vi "Start Logic-Mode dependent case 1.vi"(6 "Case name string":string, 8 "error in (no error)":errorcluster, 11 "UI queue":refnum<queue>) -> (0 "error out":errorcluster)   [LabVIEW 2013]
uses:
  Queue/Message Queue/Typedefs/Message Cluster.ctl
  Global Variables/gl_UI Ctrl Refs.vi
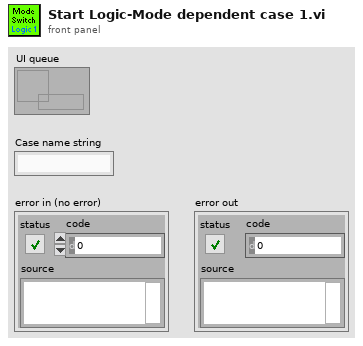
[diagram p1: front panel]
types:
  T1 = typedef "UI ctrl refs cluster.ctl" = cluster{"Top level VI path":path, "Top level VI ref":refnum<vi>, "User menu ref":refnum<k9>, "Sub Panel control":refnum<vi>, "Imaging Param Tab":refnum<vi>, "Occurrence-Start drivers":refnum<k4>, "Occurrence-Speed logging initialised":refnum<k4>, "Occurrence-XYZ stage initialised":refnum<k4>, "Exit button":refnum<vi>, "Status ind":refnum<vi>, "Return to Origin":refnum<vi>, "Speed Logging":refnum<vi>, "Time Lapse":refnum<vi>, "Live Imaging":refnum<vi>, "AOL Z Stack":refnum<vi>, "Motor Z Stack":refnum<vi>, "Funct Acq button":refnum<vi>, "Hard Shutter":refnum<vi>, "Virtual Shutter":refnum<vi>, "Laser Power":refnum<vi>, "AOL Mode":refnum<vi>, "Frame Size":refnum<vi>, "Field of View":refnum<vi>, "Dwell Time":refnum<vi>, "Zoom":refnum<vi>, "AOL Z":refnum<vi>, "Objective":refnum<vi>, "Axis":refnum<vi>, "Paths & Names":refnum<vi>, "Experiment folder path (ind.)":refnum<vi>, "Last State (Ind.)":refnum<vi>, "Laser wavelength ind (nm)":refnum<vi>, "Averages":refnum<vi>, "Angle (degrees)":refnum<vi>, "X centre":refnum<vi>, "Y centre":refnum<vi>, "Plane Mode":refnum<vi>, "# Planes":refnum<vi>, "Z Start":refnum<vi>, "Z Stop":refnum<vi>, "Z Step":refnum<vi>, "PMT 1":refnum<vi>, "PMT 2":refnum<vi>, "Stage XYZ Position":refnum<vi>, "Pockels@Z Start":refnum<vi>, "Pockels@Z Stop":refnum<vi>, "Obtain Z Start":refnum<vi>, "Obtain Z Stop":refnum<vi>, "Live stim.trig.period":refnum<vi>, "Live stim.trig.enable":refnum<vi>, "Funct. Acq. Pockels Modulation":refnum<vi>, "Enable Video Recording":refnum<vi>, "Video Record-Live Imaging":refnum<vi>, "Video Record-Funct acq":refnum<vi>, "AOL Z-stack Chirps Ready (ind)":refnum<vi>, "Center freq ind (nm)":refnum<vi>, "Logging queue (ind)":refnum<vi>, "Back aperture power (ind.)":refnum<vi>, "Power after objective (ind.)":refnum<vi>, "Switch user":refnum<vi>}
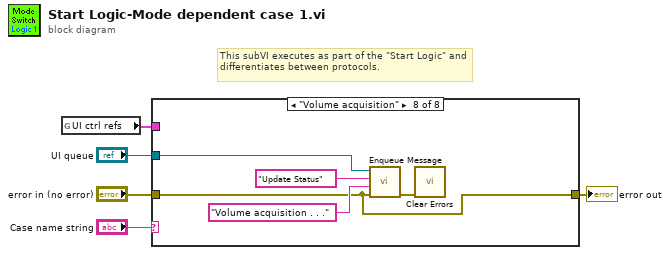
[diagram p0: block diagram]
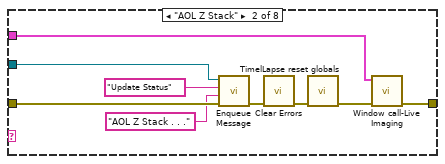
[diagram p3: hidden frame]
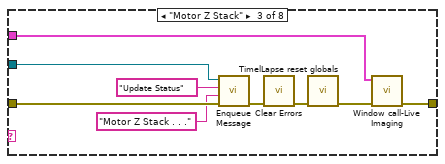
[diagram p4: hidden frame]
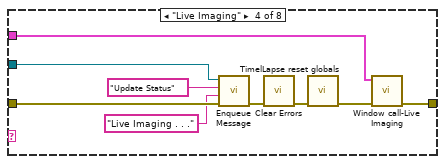
[diagram p5: hidden frame]
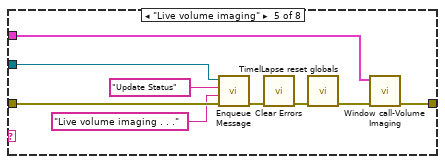
[diagram p6: hidden frame]
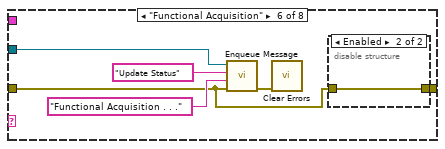
[diagram p7: hidden frame]
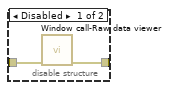
[diagram p8: hidden frame]
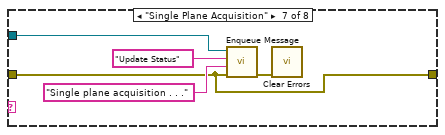
[diagram p9: hidden frame]
diagram:
  # "This subVI executes as part of the \"Start Logic\" and differentiates between protocols."
  n1 = global read "gl_UI Ctrl Refs.vi" "UI ctrl refs"() -> (w2:T1)
  n2 = case shown="\"Volume acquisition\"" "Case name string" {
    tunnel: "error in (no error)" -> [w6 w15 w24 w33 w42 w44 w52 w57]
    tunnel: "UI queue" -> [_ w14 w23 w32 w41 w48 w56 w61]
    tunnel: w2 -> [_ w8 w17 w26 w35 _ _ _]
    tunnel: [w6 w7 w16 w25 w34 w43 w52 w57] -> w1
    frame Default {
    }
    frame "AOL Z Stack" {
      n3 = call "Enqueue Message.vi"("error in (no error)"=w15, "Message Data"="AOL Z Stack . . ." ("Acquiring and Logging..."), "Message"="Update Status", "Queue"=w14) -> ("error out"=w12:errorcluster)  [unwired: 6 in, 1 out]
      n4 = call <vilib>:"Clear Errors.vi"("error in (no error)"=w12) -> ("error out"=w10:errorcluster)  [unwired: 6 in]
      n5 = call "TimelLapse reset globals.vi"("error in (no error)"=w10) -> ("error out"=w9:errorcluster)  [unwired: 10 in]
      n6 = call "Window call-Live Imaging.vi"("error in (no error)"=w9, "UI ctrl refs"=w8) -> ("error out"=w7:errorcluster)  [unwired: 9 in]
    }
    frame "Motor Z Stack" {
      n7 = call "Enqueue Message.vi"("error in (no error)"=w24, "Message Data"="Motor Z Stack . . ." ("Acquiring and Logging..."), "Message"="Update Status", "Queue"=w23) -> ("error out"=w21:errorcluster)  [unwired: 6 in, 1 out]
      n8 = call <vilib>:"Clear Errors.vi"("error in (no error)"=w21) -> ("error out"=w19:errorcluster)  [unwired: 6 in]
      n9 = call "TimelLapse reset globals.vi"("error in (no error)"=w19) -> ("error out"=w18:errorcluster)  [unwired: 10 in]
      n10 = call "Window call-Live Imaging.vi"("error in (no error)"=w18, "UI ctrl refs"=w17) -> ("error out"=w16:errorcluster)  [unwired: 9 in]
    }
    frame "Live Imaging" {
      n11 = call "Enqueue Message.vi"("error in (no error)"=w33, "Message Data"="Live Imaging . . ." ("Acquiring and Logging..."), "Message"="Update Status", "Queue"=w32) -> ("error out"=w30:errorcluster)  [unwired: 6 in, 1 out]
      n12 = call <vilib>:"Clear Errors.vi"("error in (no error)"=w30) -> ("error out"=w28:errorcluster)  [unwired: 6 in]
      n13 = call "TimelLapse reset globals.vi"("error in (no error)"=w28) -> ("error out"=w27:errorcluster)  [unwired: 10 in]
      n14 = call "Window call-Live Imaging.vi"("error in (no error)"=w27, "UI ctrl refs"=w26) -> ("error out"=w25:errorcluster)  [unwired: 9 in]
    }
    frame "Live volume imaging" {
      n15 = call "Enqueue Message.vi"("error in (no error)"=w42, "Message Data"="Live volume imaging . . ." ("Acquiring and Logging..."), "Message"="Update Status", "Queue"=w41) -> ("error out"=w39:errorcluster)  [unwired: 6 in, 1 out]
      n16 = call <vilib>:"Clear Errors.vi"("error in (no error)"=w39) -> ("error out"=w37:errorcluster)  [unwired: 6 in]
      n17 = call "TimelLapse reset globals.vi"("error in (no error)"=w37) -> ("error out"=w36:errorcluster)  [unwired: 10 in]
      n18 = call "Window call-Volume Imaging.vi"("error in (no error)"=w36, "UI ctrl refs"=w35) -> ("error out"=w34:errorcluster)  [unwired: 9 in]
    }
    frame "Functional Acquisition" {
      n19 = call "Enqueue Message.vi"("error in (no error)"=w44, "Message Data"="Functional Acquisition . . ." ("Acquiring and Logging..."), "Message"="Update Status", "Queue"=w48) -> ("error out"=w46:errorcluster)  [unwired: 6 in, 1 out]
      n20 = call <vilib>:"Clear Errors.vi"("error in (no error)"=w46) -> ()  [unwired: 6 in, 1 out]
      n21 = disable-structure shown="Enabled" {
        disable-tunnel: w44 -> [w50 w51]
        disable-tunnel: [w49 w51] -> w43
        frame Disabled {
          n22 = call "Window call-Raw data viewer.vi"("error in (no error)"=w50) -> ("error out"=w49:errorcluster)  [unwired: 10 in]
        }
        frame Enabled {
        }
      }
    }
    frame "Single Plane Acquisition" {
      n23 = call "Enqueue Message.vi"("error in (no error)"=w52, "Message Data"="Single plane acquisition . . ." ("Acquiring and Logging..."), "Message"="Update Status", "Queue"=w56) -> ("error out"=w54:errorcluster)  [unwired: 6 in, 1 out]
      n24 = call <vilib>:"Clear Errors.vi"("error in (no error)"=w54) -> ()  [unwired: 6 in, 1 out]
    }
    frame "Volume acquisition" {
      n25 = call "Enqueue Message.vi"("error in (no error)"=w57, "Message Data"="Volume acquisition . . ." ("Acquiring and Logging..."), "Message"="Update Status", "Queue"=w61) -> ("error out"=w59:errorcluster)  [unwired: 6 in, 1 out]
      n26 = call <vilib>:"Clear Errors.vi"("error in (no error)"=w59) -> ()  [unwired: 6 in, 1 out]
    }
  }
  "error out" <- w1
